vi "Configure.vi"(8 "error in (no error)":errorcluster, 11 "Temp Monitor in":refnum<class "Standard Measurement.lvclass">) -> (0 "error out":errorcluster, 3 "Temp Monitor out":refnum<class "Standard Measurement.lvclass">)   [LabVIEW 2026, in "Standard Measurement Plugin.lvlib" / "Standard Measurement.lvclass"]
doc: "Override configure.vi to setup any parameters for a measurement before acquiring.\n\nConfigure.vi is called by the 'Initialize Measurement Actor Core.vi,' which executes before Actor Core of the root measurement class. The root configure method populates the basic Measurement UI with information such as the hardware device in use and the name of the measurement. The base configure method calls 'Acquire.vi' once execution is complete. If beginning a recurring acquisition, it reset the iteration count to zero."
uses:
  Standard Measurement.lvclass
  framework/Measurement Actor/Measurement.lvclass
  Standard Measurement.lvclass/Standard Measurement.ctl
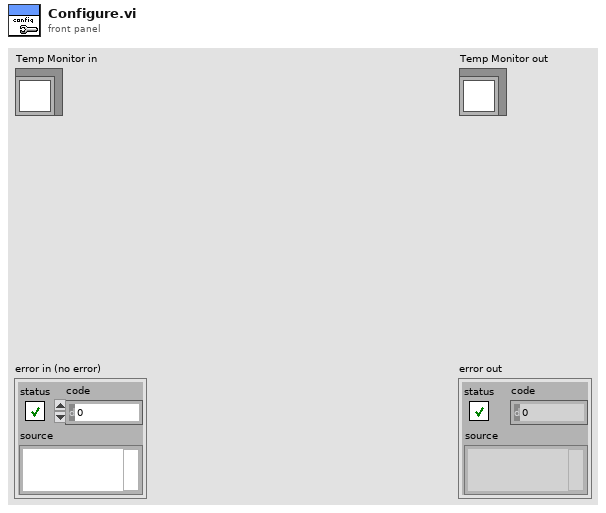
[diagram p1: front panel]
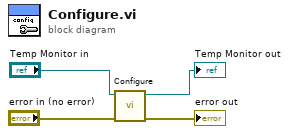
[diagram p0: block diagram]
diagram:
  n1 = call-parent "Configure.vi"("error in (no error)"="error in (no error)", "Measurement in"="Temp Monitor in") -> ("error out"=→"error out":errorcluster, "Measurement out"=→"Temp Monitor out":refnum<class "Standard Measurement.lvclass">)  [unwired: 8 in]
